vi "PH_Cont-601k_PSU.Dev Set Mode.vi"(0 "VI in":refnum<vi>, 5 "error in (no error)":errorcluster) -> (14 "VI out":refnum<vi>, 18 "Device Error out":errorcluster, 19 "error out":errorcluster)   [LabVIEW 2014, in "PH_Cont-601k_PSU.lvlib"]
uses:
  PH_Cont-601k_PSU.lvlib
  instr.lib/pu601k/Continuum PU610K.lvlib
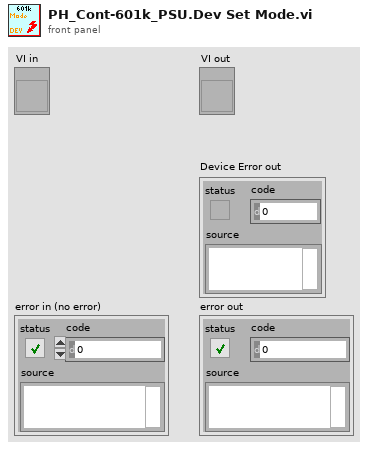
[diagram p1: front panel]
types:
  T1 = typedef "PH_Cont-601k_PSU.lvlib/PH_Cont-601k_PSU.i attribute.ctl" = cluster{"GUI Refs":T2, "Interlock":bool, "Service ID applied Voltage":i32, "Device Settings":cluster{"Configuration":T3, "Flash Interval [s]":dbl, "Mode":T4, "Voltage [V]":u16, "Charge":bool, "VISA resource name":refnum<visa-resource-name>}, "Readyness":T5, "Information":cluster{"VISA resource name":refnum<visa-resource-name>, "Tagname Power On":string, "Interlock":cluster{"Instance":string, "Tagname":string}, "Limits [V]":cluster{"Lower":dbl, "Upper":dbl}, "Tagname PSU On":string}, "R2S":bool, "Charge is allowed":bool}
  T2 = typedef "PH_Cont-601k_PSU.lvlib/PH_Cont-601k_PSU.GUI Refs.ctl" = cluster{"Power On":refnum<vi>, "Hard- and Software":refnum<vi>, "Device Status":refnum<vi>, "Device Error":refnum<vi>, "Configuration":refnum<vi>, "Flash Interval [s]":refnum<vi>, "Interlock":refnum<vi>, "Interlock Indicator":refnum<vi>, "Voltage [V]":refnum<vi>, "Readyness":refnum<vi>, "Mode":refnum<vi>, "Reset Error":refnum<vi>, "Expert working":refnum<vi>, "Charge":refnum<vi>, "PSU On":refnum<vi>}
  T3 = typedef "PH_Cont-601k_PSU.lvlib/PH_Cont-601k_PSU.Configuration.ctl" = u16
  T4 = typedef "PH_Cont-601k_PSU.lvlib/PH_Cont-601k_PSU.Mode.ctl" = enum32{"STOP", "STANDBY", "READY", "EMISSION", "ERROR"}
  T5 = typedef "PH_Cont-601k_PSU.lvlib/PH_Cont-601k_PSU.Readyness.ctl" = cluster{"Program":T6, "Device":T7}
  T6 = typedef "PH_Cont-601k_PSU.lvlib/PH_Cont-601k_PSU.Readyness Program.ctl" = enum32{"OFF", "POWER", "INTERLOCK"}
  T7 = typedef "PH_Cont-601k_PSU.lvlib/PH_Cont-601k_PSU.Readyness Device.ctl" = enum32{"OFF", "CONNECTING", "CONNECTED", "OPERATING", "EOC", "ERROR"}
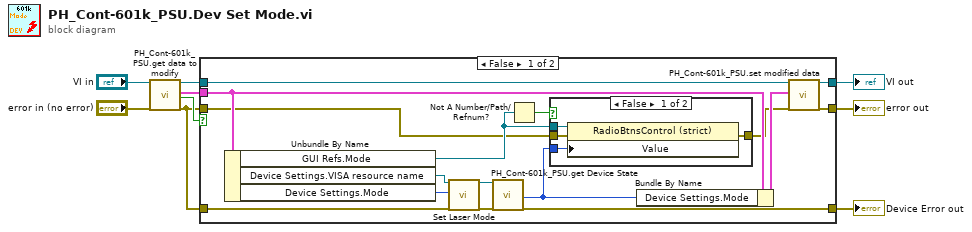
[diagram p0: block diagram]
diagram:
  n1 = call "PH_Cont-601k_PSU.get data to modify.vi"("i ref in"="VI in", "error in (no error)"="error in (no error)") -> ("i ref out"=w5:refnum<vi>, "i attribute"=w9:T1, "timed out"=w3:bool, "error out"=w1:errorcluster)  [unwired: 14 in]
  n2 = case shown="False" w3 {
    tunnel: w9 -> [w20 _]
    tunnel: w1 -> [w11 w32]
    tunnel: [w16 w31] -> w7
    tunnel: [w23 w32] -> w6
    tunnel: w5 -> [w22 w33]
    tunnel: [w21 w33] -> w4
    tunnel: w1 -> [w10 w31]
    frame False {
      n3 = Unbundle By Name(w20) -> ("GUI Refs.Mode"=w12:refnum<vi>, "Device Settings.VISA resource name"=w25:refnum<visa-resource-name>, "Device Settings.Mode"=w24:T4)
      n4 = call "Set Laser Mode.vi"("VISA resource name"=w25, "Mode"=w24, "error in"=w10) -> ("VISA resource name out"=w17:refnum<visa-resource-name>, "error out"=w18:errorcluster)  [unwired: 15 in]
      n5 = call "PH_Cont-601k_PSU.get Device State.vi"("VISA Refnum in"=w17, "Device Error in"=w18) -> ("Mode"=w14:T4, "Device Error out"=w16:errorcluster)  [unwired: 9 in, 7 out]
      n6 = Not A Number/Path/Refnum?(number/path/refnum=w12) -> (NaN/Path/Refnum?=w13:bool)
      n7 = case shown="False" w13 {
        tunnel: w11 -> [w29 w30]
        tunnel: [w28 w30] -> w15
        tunnel: w12 -> [w27 _]
        tunnel: w14 -> [w26 _]
        frame False {
          n8 = property class="RadioBtnsControl (strict)"(reference=w27, error in=w29, "Value"=w26) -> (error out=w28:errorcluster)  [unwired: 1 out]
        }
        frame True {
        }
      }
      n9 = Bundle By Name(cluster=w20, "Device Settings.Mode"=w14) -> (w19:T1)
      n10 = call "PH_Cont-601k_PSU.set modified data.vi"("i ref in"=w22, "i attribute"=w19, "error in (no error)"=w15) -> ("i ref out"=w21:refnum<vi>, "error out"=w23:errorcluster)  [unwired: 15 in]
    }
    frame True {
    }
  }
  "error out" <- w6
  "VI out" <- w4
  "Device Error out" <- w7
